vi "Online_target.vi"   [LabVIEW 2021]
uses:
  Model_Updating_Classes/DROPBEAR_Model_Updating/DROPBEAR_Model_Updating.lvclass
  Model_Updating_Classes/MOCKBEAR/MOCKBEAR.lvclass
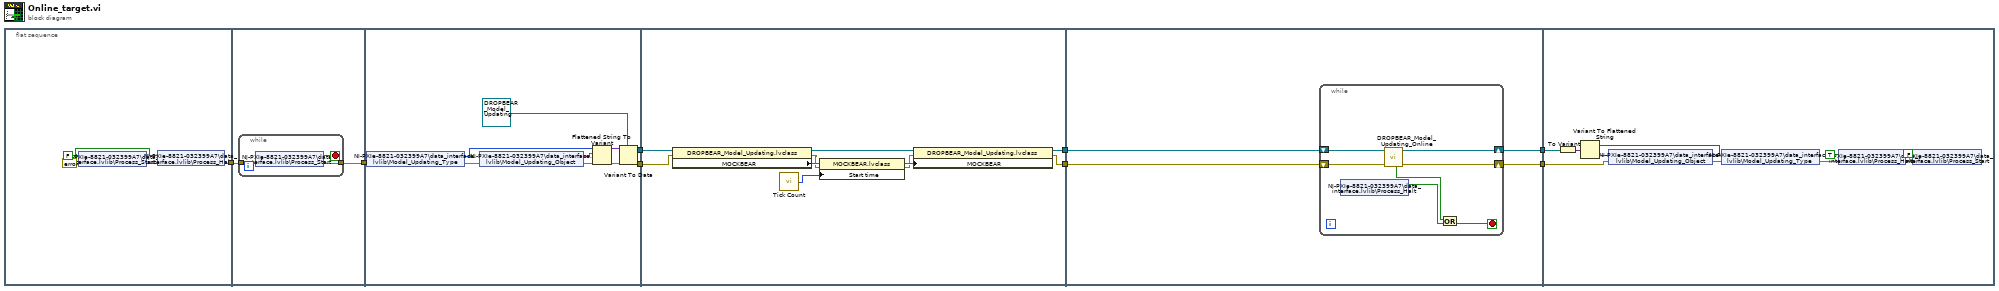
[diagram p0: block diagram]
diagram:
  n1 = flat-sequence {
    tunnel: [w10] -> w6
    tunnel: w6 -> [w14]
    tunnel: [w13] -> w5
    tunnel: [w20] -> w4
    tunnel: [w21] -> w2
    tunnel: w5 -> [w19]
    tunnel: w4 -> [w28]
    tunnel: [w31] -> w3
    tunnel: w2 -> [w32]
    tunnel: [w30] -> w1
    tunnel: w3 -> [w41]
    tunnel: [w40] -> w8
    tunnel: w1 -> [w39]
    tunnel: [w38] -> w7
    tunnel: w8 -> [w58]
    tunnel: w7 -> [w51]
    frame #0 {
      w9 = FALSE ("Process_Start")
      n2 = shared-variable "NI-PXIe-8821-032399A7\\data_interface.lvlib\\Process_Start"(w9, error in=errorcluster {"status"=FALSE, "code"=0, "source"=""} ("error in (no error)")) -> (error out=w11:errorcluster)
      n3 = shared-variable "NI-PXIe-8821-032399A7\\data_interface.lvlib\\Process_Halt"(w9, error in=w11) -> (error out=w10:errorcluster)
    }
    frame #1 {
      n4 = while {
        tunnel: w14 -> [w16]
        tunnel: [w15] -> w13
        stop <- w17 stop-if-true
        n5 = shared-variable "NI-PXIe-8821-032399A7\\data_interface.lvlib\\Process_Start"(error in=w16) -> (w17:bool, error out=w15:errorcluster)
      }
    }
    frame #2 {
      n6 = shared-variable "NI-PXIe-8821-032399A7\\data_interface.lvlib\\Model_Updating_Type"(error in=w19) -> (w25:i16[], error out=w22:errorcluster)
      n7 = shared-variable "NI-PXIe-8821-032399A7\\data_interface.lvlib\\Model_Updating_Object"(error in=w22) -> (w24:string, error out=w23:errorcluster)
      n8 = Flattened String To Variant(4:w23, 6:w24, 7:w25) -> (0:w27:errorcluster, 3:w26:variant)
      n9 = Variant To Data(error in=w27, type=refnum<class "DROPBEAR_Model_Updating.lvclass"> refnum ("DROPBEAR_Model_Updating.lvclass"), Variant=w26) -> (data=w20:refnum<class "DROPBEAR_Model_Updating.lvclass">, error out=w21:errorcluster)
    }
    frame #3 {
      n10 = property class="DROPBEAR_Model_Updating.lvclass"(reference=w28, error in=w32) -> (reference out=w35:refnum<class "DROPBEAR_Model_Updating.lvclass">, error out=w29:errorcluster, "MOCKBEAR"=w37:refnum<class "MOCKBEAR.lvclass">)
      n11 = call "Tick Count"() -> ("Tick Count(uSec)"=w34:u32)
      n12 = property class="MOCKBEAR.lvclass"(reference=w37, error in=w29, "Start time"=w34) -> (reference out=w36:refnum<class "MOCKBEAR.lvclass">, error out=w33:errorcluster)
      n13 = property class="DROPBEAR_Model_Updating.lvclass"(reference=w35, error in=w33, "MOCKBEAR"=w36) -> (reference out=w31:refnum<class "DROPBEAR_Model_Updating.lvclass">, error out=w30:errorcluster)
    }
    frame #4 {
      n14 = while {
        shift-right: [w44] -> w40
        shift-left: w41 -> [w46]
        shift-right: [w43] -> w38
        shift-left: w39 -> [w45]
        stop <- w48 stop-if-true
        n15 = shared-variable "NI-PXIe-8821-032399A7\\data_interface.lvlib\\Process_Halt"() -> (w47:bool)  [unwired: 1 in, 1 out]
        n16 = call-dynamic "DROPBEAR_Model_Updating_Online.vi"("error in (no error)"=w45, "DROPBEAR_Model_Updating in"=w46) -> ("error out"=w43:errorcluster, "DROPBEAR_Model_Updating out"=w44:refnum<class "DROPBEAR_Model_Updating.lvclass">, "looping"=w42:bool)  [unwired: 7 in]
        n17 = Or(x=w42, y=w47) -> (x .or. y?=w48:bool)
      }
    }
    frame #5 {
      n18 = To Variant(anything=w58) -> (Variant=w53:variant)
      n19 = Variant To Flattened String(Variant=w53) -> (data string=w56:string, 1:w54:i16[])
      n20 = shared-variable "NI-PXIe-8821-032399A7\\data_interface.lvlib\\Model_Updating_Object"(w56, error in=w51) -> (error out=w55:errorcluster)
      n21 = shared-variable "NI-PXIe-8821-032399A7\\data_interface.lvlib\\Model_Updating_Type"(w54, error in=w55) -> (error out=w52:errorcluster)
      n22 = shared-variable "NI-PXIe-8821-032399A7\\data_interface.lvlib\\Process_Halt"(TRUE ("Process_Halt"), error in=w52) -> (error out=w50:errorcluster)
      n23 = shared-variable "NI-PXIe-8821-032399A7\\data_interface.lvlib\\Process_Start"(FALSE ("Process_Start"), error in=w50) -> ()  [unwired: 1 out]
    }
  }
